vi "Read configuration.vi"(8 "error in":errorcluster, 11 "CVT editor node in":refnum<class "CVT editor node.lvclass">) -> (0 "error out":errorcluster, 2 "configuration":refnum<class "NISE_CEF_serializable configuration.lvclass">, 3 "CVT editor node out":refnum<class "CVT editor node.lvclass">)   [LabVIEW 2013, in "CVT editor node.lvclass"]
uses:
  CVT editor node.lvclass
  <vilib>/NI/Configuration Framework/serializable configuration/NISE_CEF_serializable configuration.lvclass
  CVT editor node.lvclass/CVT editor node.ctl
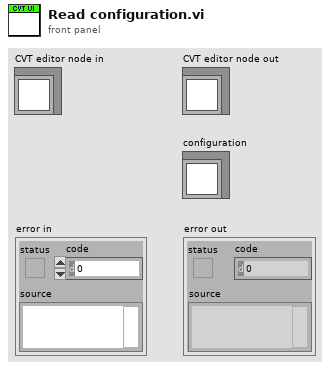
[diagram p1: front panel]
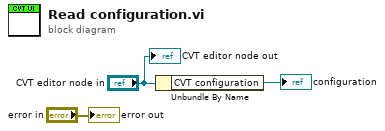
[diagram p0: block diagram]
diagram:
  n1 = Unbundle By Name("CVT editor node in") -> ("CVT configuration"=→"configuration":refnum<class "CVT configuration.lvclass">)
  "error out" <- "error in"
  "CVT editor node out" <- "CVT editor node in"
